vi "CAN Set Value.vi"(7 "BufferLength":u32, 8 "error in (no error)":errorcluster, 9 "Buffer":u32, 10 "Parameter":u8, 11 "Channel":u16) -> (0 "error out":errorcluster, 1 "Buffer out":u32, 3 "function return":u32)   [LabVIEW 2025, in "PCAN2023.lvlib"]
doc: "Configures or sets a PCAN Channel value\n\n\nTPCANStatus __stdcall CAN_SetValue(\n TPCANHandle Channel,\n TPCANParameter Parameter,\n void* Buffer,\n DWORD BufferLength);"
uses:
  PCAN2023.lvlib
  x64/PCANBasic.dll
panel:
  out "Channel out":u16
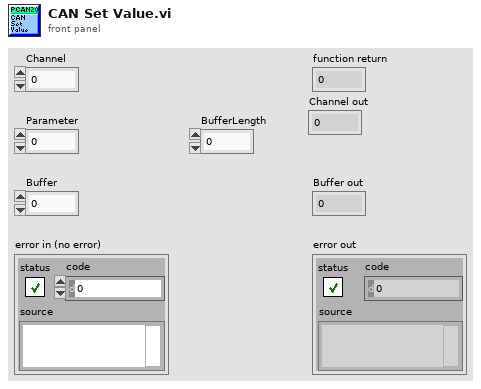
[diagram p1: front panel]
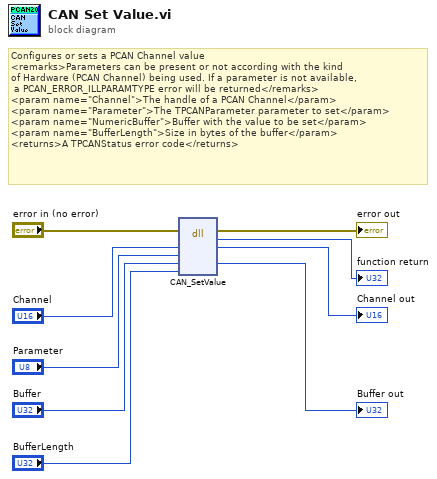
[diagram p0: block diagram]
diagram:
  # "Configures or sets a PCAN Channel value \n<remarks>Parameters can be present or not according with the kind \nof Hardware (PCAN Channel) being used. If a parameter is not available,\n a PCAN_ERROR_ILLPARAMTYPE error will be returned</remarks>\n<param name=\"Channel\">The handle of a PCAN Channel</param>\n<param name=\"Parameter\">The TPCANParameter parameter to set</param>\n<param name=\"NumericBuffer\">Buffer with the value to be set</param>\n<param name=\"BufferLength\">Size in bytes of the buffer</param>\n<returns>A TPCANStatus error code</returns>"
  n1 = dll-call lib="C:/UTP/LabView/Communication Handle/PCAN2023/x64/PCANBasic.dll" fn="CAN_SetValue"(error in="error in (no error)", "Channel"="Channel", "Parameter"="Parameter", "Buffer"="Buffer", "BufferLength"="BufferLength") -> (error out=→"error out":errorcluster, "return type"=→"function return":u32, "Channel"=→"Channel out":u16, "Buffer"=→"Buffer out":u32)  [unwired: 4 in, 1 out]
